vi "35.vi"() -> ()   [LabVIEW 2021]
uses:
  8260e4b7-20d0-4637-845c-86187f89e6fe.vi
  f9f8941c-c77f-431b-8773-34b27d578bd3.vi
  <vilib>/Comparison/Less/Less Functor/Less Functor.lvclass
  <vilib>/gmath/NI_AAL_MathFunc.lvlib
panel:
  out "size(s)":i32
  out "sorted array":i32[](array[numeric])
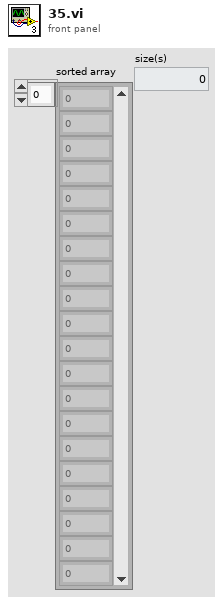
[diagram p1: front panel]
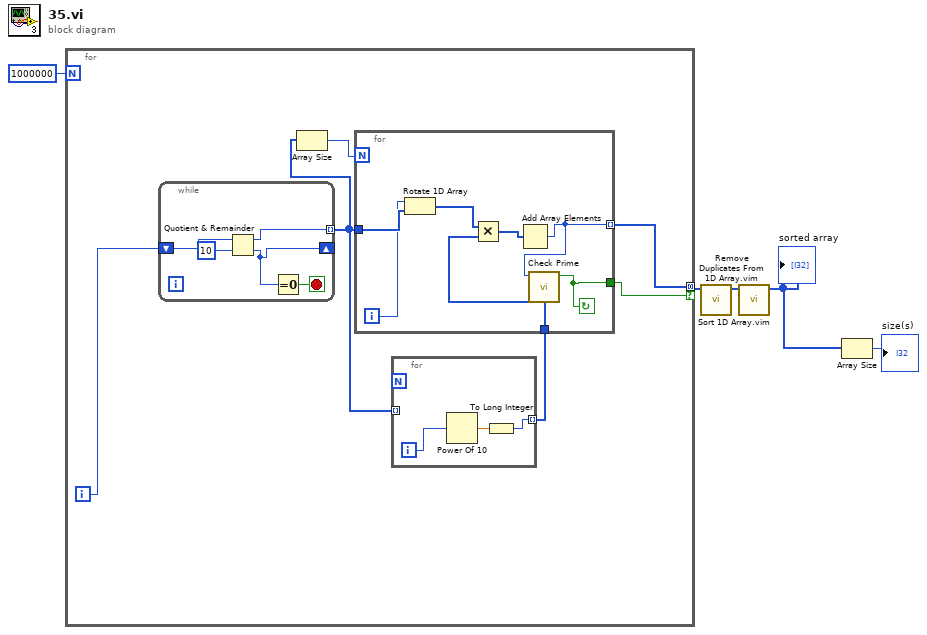
[diagram p0: block diagram]
diagram:
  n1 = for {
    N: 1000000 -> [_]
    tunnel: [w7] -> w4 mode=concatenating if=w6
    i -> [w11]
    n2 = while {
      tunnel: [w23] -> w8 mode=indexing
      shift-right: [w22] -> _
      shift-left: w11 -> [w26]
      stop <- w24 stop-if-true
      n3 = Quotient & Remainder(x=w26, y=10) -> (x-y*floor(x/y)=w23:i32, floor(x/y)=w22:i32)
      n4 = Equal To 0?(x=w22) -> (x = 0?=w24:bool)
    }
    n5 = Array Size(array=w8) -> (size(s)=w9:i32)
    n6 = for {
      tunnel: w8 -> [_] mode=indexing
      tunnel: [w19] -> w10 mode=indexing
      i -> [w21]
      n7 = Power Of 10(x=w21) -> (10^x=w20:dbl)
      n8 = To Long Integer(number=w20) -> (32bit integer=w19:i32)
    }
    n9 = for {
      N: w9 -> [_]
      tunnel: w8 -> [w18]
      tunnel: w10 -> [w17]
      tunnel: [w13] -> w7 mode=indexing
      tunnel: [w12] -> w6
      i -> [w14]
      stop <- w12 continue-if-true
      n10 = Rotate 1D Array(1:w18, 2:w14) -> (0:w16:i32[])
      n11 = Multiply(x=w16, y=w17) -> (x*y=w15:i32[])
      n12 = Add Array Elements(numeric array=w15) -> (sum=w13:i32)
      n13 = call <vilib>:"Check Prime.vi"("n"=w13) -> ("prime?"=w12:bool)  [unwired: 10 in]
    }
  }
  n14 = call "Remove Duplicates From 1D Array.vim"("array"=w4) -> ("array with duplicates removed"=w3:i32[])  [unwired: 10 in]
  n15 = call "Sort 1D Array.vim"("unsorted array"=w3) -> ("sorted array"=w2:i32[])  [unwired: 10 in]
  "sorted array" <- w2
  n16 = Array Size(array=w2) -> (size(s)=→"size(s)":i32)
